vi "IT6322Control.vi"(9 "通道1":dbl, 10 "VISA resource name":refnum<visa-resource-name> caption="VISA资源名称", 11 "Sequence Context In":refnum<k7>) -> (0 "error out":errorcluster, 1 "输出":dbl, 3 "Report Text":string)   [LabVIEW 2018]
uses:
  <vilib>/Instr/_visa.llb/VISA Configure Serial Port (Instr).vi
panel:
  out "输出 3":dbl
  out "输出 2":dbl
  in  "通道3":dbl
  in  "通道2":dbl
  in  "功能":T1(ring)
  in  "error in (no error)":errorcluster caption="错误输入（无错误）"
  # "IT6322 CONTROL"
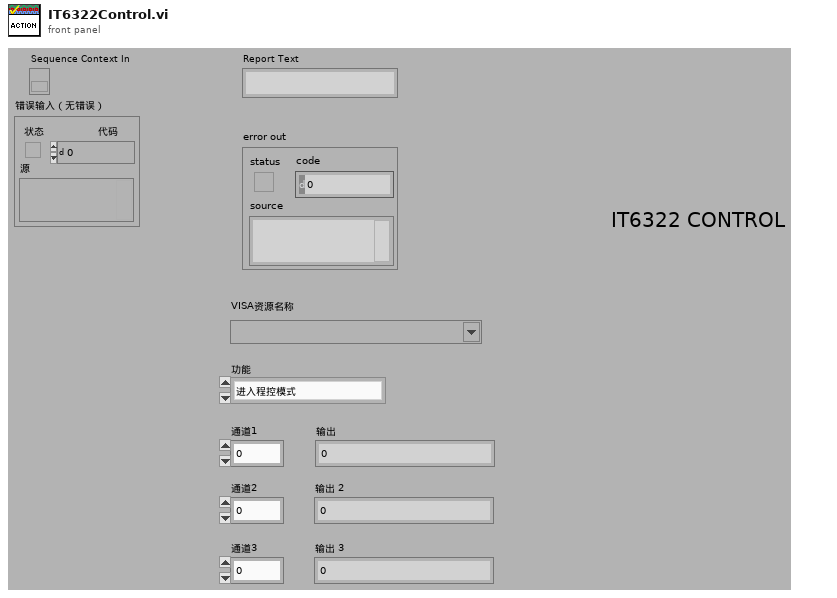
[diagram p1: front panel]
types:
  T1 = enum16{"进入程控模式", "输出ON", "输出OFF", "设置电压", "设置电流", "读取电压", "读取电流"}
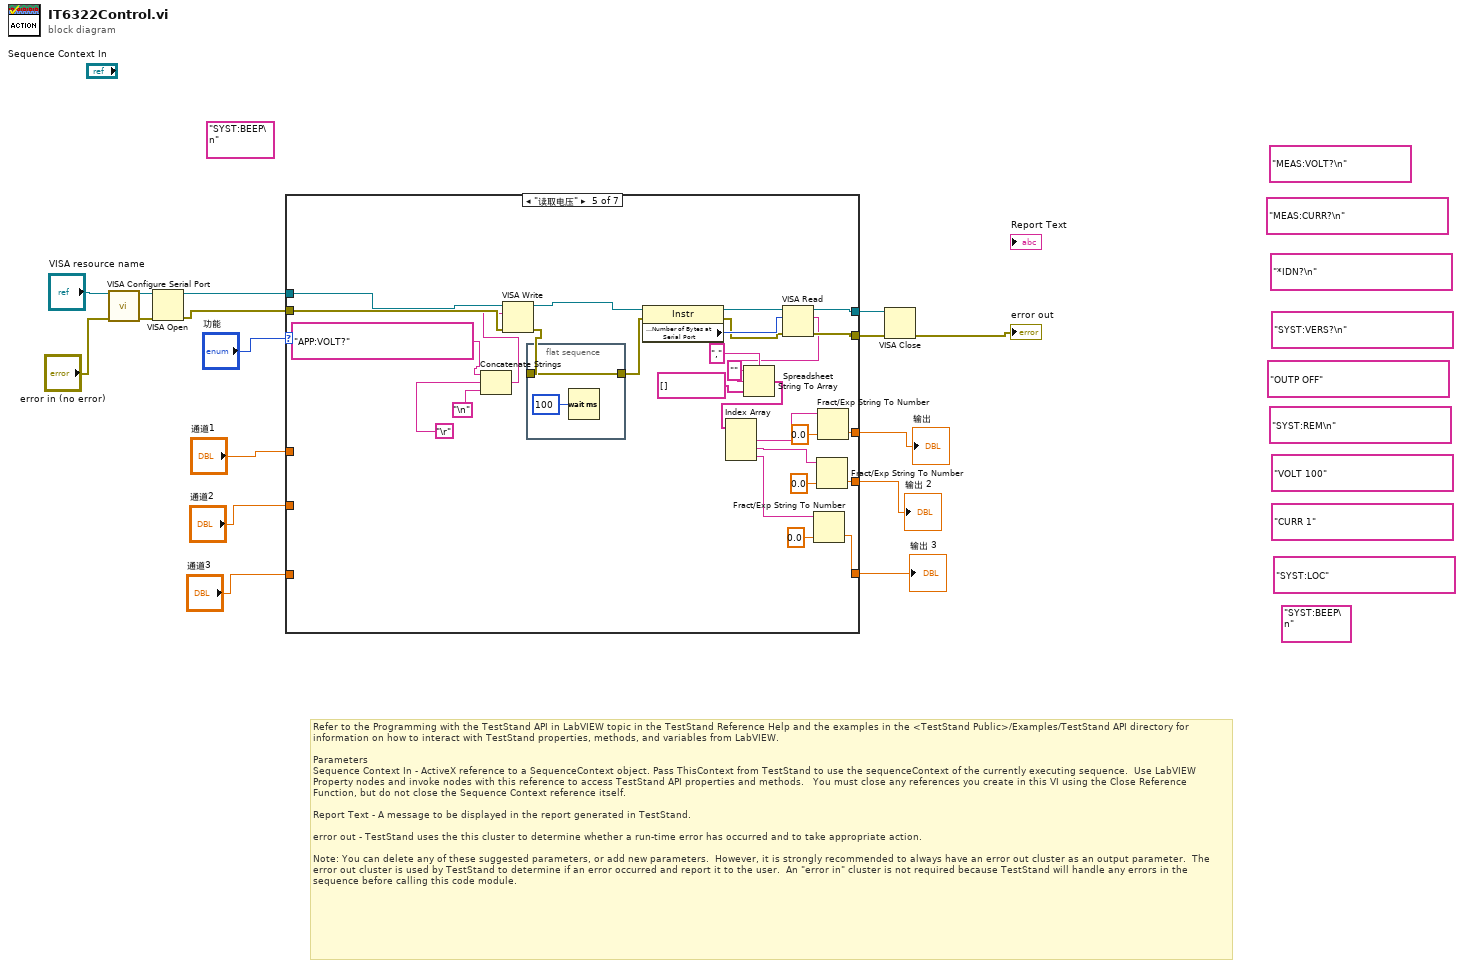
[diagram p0: block diagram]
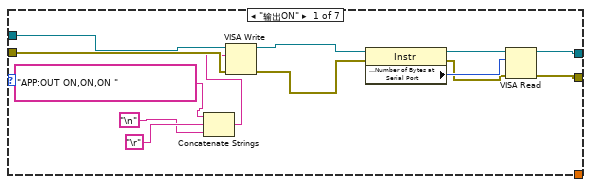
[diagram p2: hidden frame]
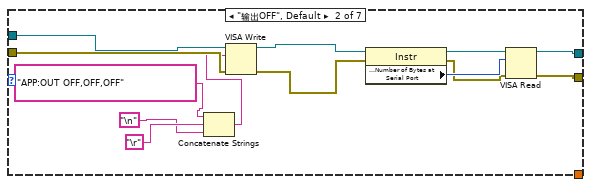
[diagram p3: hidden frame]
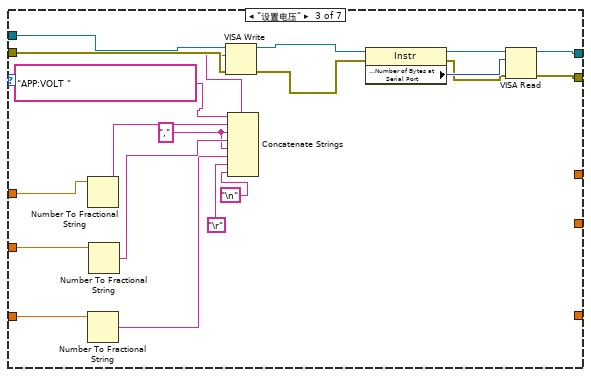
[diagram p4: hidden frame]
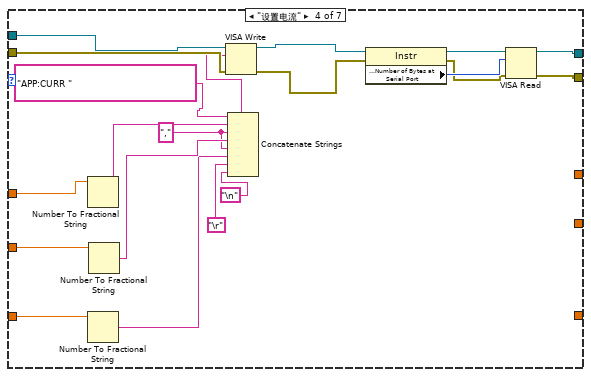
[diagram p5: hidden frame]
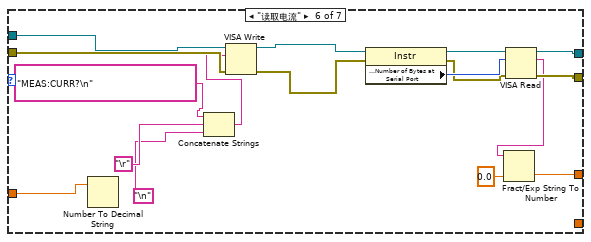
[diagram p6: hidden frame]
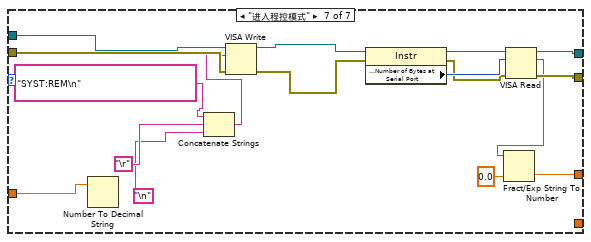
[diagram p7: hidden frame]
diagram:
  (unwired) "SYST:LOC" ("写入缓冲区")
  (unwired) "CURR 1" ("写入缓冲区")
  (unwired) "VOLT 100" ("写入缓冲区")
  (unwired) "OUTP OFF" ("写入缓冲区")
  (unwired) "SYST:REM\n" ("写入缓冲区")
  (unwired) "SYST:VERS?\n" ("写入缓冲区")
  (unwired) "*IDN?\n" ("写入缓冲区")
  (unwired) "MEAS:CURR?\n" ("写入缓冲区")
  (unwired) "MEAS:VOLT?\n" ("写入缓冲区")
  (unwired) "SYST:BEEP\n" ("写入缓冲区")
  (unwired) "SYST:BEEP\n" ("写入缓冲区")
  # "Refer to the Programming with the TestStand API in LabVIEW topic in the TestStand Reference Help and the examples in the <TestStand Public>/Examples/TestStand API directory for information on how to interact with TestStand properties, methods, and variables from LabVIEW.\n\nParameters\nSequence Context In - ActiveX reference to a SequenceContext object. Pass ThisContext from TestStand to use the sequenceContext of the currently executing sequence.  Use LabVIEW Property nodes and invoke nodes with this reference to access TestStand API properties and methods.   You must close any references you create in this VI using the Close Reference Function, but do not close the Sequence Context reference itself.\n\nReport Text - A message to be displayed in the report generated in TestStand. \n\nerror out - TestStand uses the this cluster to determine whether a run-time error has occurred and to take appropriate action.  \n\nNote: You can delete any of these suggested parameters, or add new parameters.  However, it is strongly recommended to always have an error out cluster as an output parameter.  The error out cluster is used by TestStand to determine if an error occurred and report it to the user.  An \"error in\" cluster is not required because TestStand will handle any errors in the sequence before calling this code module."
  n1 = call-poly "VISA Configure Serial Port"("VISA resource name"="VISA resource name", "error in (no error)"="error in (no error)") -> ("VISA resource name out"=w14:refnum<visa-resource-name>, "error out"=w15:errorcluster)  [unwired: 12 in]
  n2 = VISA Open(error in (no error)=w15, VISA resource name=w14) -> (VISA resource name=w13:refnum<visa-resource-name>, error out=w12:errorcluster)  [unwired: 3 in]
  n3 = case shown="\"读取电压\"" "功能" {
    tunnel: w13 -> [w29 w42 w62 w82 w110 w129 w146]
    tunnel: w12 -> [w28 w41 w61 w81 w109 w128 w145]
    tunnel: [w20 w33 w53 w73 w101 w120 w137] -> w10
    tunnel: [w19 w32 w52 w72 w100 w119 w136] -> w9
    tunnel: "通道1" -> [_ _ w48 w68 _ w116 w133]
    tunnel: [_ _ _ _ w97 w113 w130] -> w5
    tunnel: "通道2" -> [_ _ w47 w67 _ _ _]
    tunnel: "通道3" -> [_ _ w46 w66 _ _ _]
    tunnel: [_ _ _ _ w86 _ _] -> w2
    tunnel: [_ _ _ _ w85 _ _] -> w1
    frame "输出ON" {
      n4 = Concatenate Strings("APP:OUT ON,ON,ON " ("写入缓冲区"), "\r", "\n") -> (w23:string)
      n5 = VISA Write(VISA resource name=w29, write buffer=w23, error in (no error)=w28) -> (VISA resource name out=w27:refnum<visa-resource-name>, error out=w17:errorcluster)  [unwired: 1 out]
      n6 = property class="Instr"(reference=w27, error in=w17) -> (reference out=w26:refnum<visa-resource-name>, error out=w18:errorcluster, "Serial Settings:Number of Bytes at Serial Port"=w25:u32)
      n7 = VISA Read(VISA resource name=w26, byte count=w25, error in (no error)=w18) -> (VISA resource name out=w20:refnum<visa-resource-name>, error out=w19:errorcluster)  [unwired: 2 out]
    }
    frame "输出OFF", Default {
      n8 = Concatenate Strings("APP:OUT OFF,OFF,OFF" ("写入缓冲区"), "\r", "\n") -> (w36:string)
      n9 = VISA Write(VISA resource name=w42, write buffer=w36, error in (no error)=w41) -> (VISA resource name out=w40:refnum<visa-resource-name>, error out=w30:errorcluster)  [unwired: 1 out]
      n10 = property class="Instr"(reference=w40, error in=w30) -> (reference out=w39:refnum<visa-resource-name>, error out=w31:errorcluster, "Serial Settings:Number of Bytes at Serial Port"=w38:u32)
      n11 = VISA Read(VISA resource name=w39, byte count=w38, error in (no error)=w31) -> (VISA resource name out=w33:refnum<visa-resource-name>, error out=w32:errorcluster)  [unwired: 2 out]
    }
    frame "设置电压" {
      w44 = "," ("string")
      n12 = Number To Fractional String(number=w48) -> (F-format string=w49:string)  [unwired: 3 in]
      n13 = Number To Fractional String(number=w46) -> (F-format string=w43:string)  [unwired: 3 in]
      n14 = Number To Fractional String(number=w47) -> (F-format string=w45:string)  [unwired: 3 in]
      n15 = Concatenate Strings("APP:VOLT " ("写入缓冲区"), w49, w44, w45, w44, w43, "\r", "\n") -> (w56:string)
      n16 = VISA Write(VISA resource name=w62, write buffer=w56, error in (no error)=w61) -> (VISA resource name out=w60:refnum<visa-resource-name>, error out=w50:errorcluster)  [unwired: 1 out]
      n17 = property class="Instr"(reference=w60, error in=w50) -> (reference out=w59:refnum<visa-resource-name>, error out=w51:errorcluster, "Serial Settings:Number of Bytes at Serial Port"=w58:u32)
      n18 = VISA Read(VISA resource name=w59, byte count=w58, error in (no error)=w51) -> (VISA resource name out=w53:refnum<visa-resource-name>, error out=w52:errorcluster)  [unwired: 2 out]
    }
    frame "设置电流" {
      w64 = "," ("string")
      n19 = Number To Fractional String(number=w68) -> (F-format string=w69:string)  [unwired: 3 in]
      n20 = Number To Fractional String(number=w66) -> (F-format string=w63:string)  [unwired: 3 in]
      n21 = Number To Fractional String(number=w67) -> (F-format string=w65:string)  [unwired: 3 in]
      n22 = Concatenate Strings("APP:CURR " ("写入缓冲区"), w69, w64, w65, w64, w63, "\r", "\n") -> (w76:string)
      n23 = VISA Write(VISA resource name=w82, write buffer=w76, error in (no error)=w81) -> (VISA resource name out=w80:refnum<visa-resource-name>, error out=w70:errorcluster)  [unwired: 1 out]
      n24 = property class="Instr"(reference=w80, error in=w70) -> (reference out=w79:refnum<visa-resource-name>, error out=w71:errorcluster, "Serial Settings:Number of Bytes at Serial Port"=w78:u32)
      n25 = VISA Read(VISA resource name=w79, byte count=w78, error in (no error)=w71) -> (VISA resource name out=w73:refnum<visa-resource-name>, error out=w72:errorcluster)  [unwired: 2 out]
    }
    frame "读取电压" {
      n26 = Concatenate Strings("APP:VOLT?" ("写入缓冲区"), "\r", "\n") -> (w104:string)
      n27 = VISA Write(VISA resource name=w110, write buffer=w104, error in (no error)=w109) -> (VISA resource name out=w108:refnum<visa-resource-name>, error out=w95:errorcluster)  [unwired: 1 out]
      n28 = flat-sequence {
        tunnel: [w112] -> w96
        tunnel: w95 -> [w112]
        frame #0 {
          n29 = Wait (ms)(milliseconds to wait=u32 100) -> ()  [unwired: 1 out]
        }
      }
      n30 = property class="Instr"(reference=w108, error in=w96) -> (reference out=w107:refnum<visa-resource-name>, error out=w99:errorcluster, "Serial Settings:Number of Bytes at Serial Port"=w106:u32)
      n31 = VISA Read(VISA resource name=w107, byte count=w106, error in (no error)=w99) -> (VISA resource name out=w101:refnum<visa-resource-name>, read buffer=w84:string, error out=w100:errorcluster)  [unwired: 1 out]
      n32 = Spreadsheet String To Array(delimiter (Tab)=",", format string="", spreadsheet string=w84, array type (2D Dbl)=string[] []) -> (array=w90:string[])
      n33 = Index Array(array=w90) -> (element #1=w89:string, element #2=w88:string, element #3=w87:string)  [unwired: 3 in]
      n34 = Fract/Exp String To Number(string=w87, default (0 dbl)=0.0 ("默认(0 I32)")) -> (number=w85:dbl)  [unwired: 2 in, 1 out]
      n35 = Fract/Exp String To Number(string=w88, default (0 dbl)=0.0 ("默认(0 I32)")) -> (number=w86:dbl)  [unwired: 2 in, 1 out]
      n36 = Fract/Exp String To Number(string=w89, default (0 dbl)=0.0 ("默认(0 I32)")) -> (number=w97:dbl)  [unwired: 2 in, 1 out]
    }
    frame "读取电流" {
      n37 = Number To Decimal String(number=w116) -> ()  [unwired: 1 in, 1 out]
      n38 = Concatenate Strings("MEAS:CURR?\n" ("写入缓冲区"), "\r", "\n") -> (w123:string)
      n39 = VISA Write(VISA resource name=w129, write buffer=w123, error in (no error)=w128) -> (VISA resource name out=w127:refnum<visa-resource-name>, error out=w117:errorcluster)  [unwired: 1 out]
      n40 = property class="Instr"(reference=w127, error in=w117) -> (reference out=w126:refnum<visa-resource-name>, error out=w118:errorcluster, "Serial Settings:Number of Bytes at Serial Port"=w125:u32)
      n41 = VISA Read(VISA resource name=w126, byte count=w125, error in (no error)=w118) -> (VISA resource name out=w120:refnum<visa-resource-name>, read buffer=w115:string, error out=w119:errorcluster)  [unwired: 1 out]
      n42 = Fract/Exp String To Number(string=w115, default (0 dbl)=0.0 ("默认(0 I32)")) -> (number=w113:dbl)  [unwired: 2 in, 1 out]
    }
    frame "进入程控模式" {
      n43 = Number To Decimal String(number=w133) -> ()  [unwired: 1 in, 1 out]
      n44 = Concatenate Strings("SYST:REM\n" ("写入缓冲区"), "\r", "\n") -> (w140:string)
      n45 = VISA Write(VISA resource name=w146, write buffer=w140, error in (no error)=w145) -> (VISA resource name out=w144:refnum<visa-resource-name>, error out=w134:errorcluster)  [unwired: 1 out]
      n46 = property class="Instr"(reference=w144, error in=w134) -> (reference out=w143:refnum<visa-resource-name>, error out=w135:errorcluster, "Serial Settings:Number of Bytes at Serial Port"=w142:u32)
      n47 = VISA Read(VISA resource name=w143, byte count=w142, error in (no error)=w135) -> (VISA resource name out=w137:refnum<visa-resource-name>, read buffer=w132:string, error out=w136:errorcluster)  [unwired: 1 out]
      n48 = Fract/Exp String To Number(string=w132, default (0 dbl)=0.0 ("默认(0 I32)")) -> (number=w130:dbl)  [unwired: 2 in, 1 out]
    }
  }
  "输出" <- w5
  "输出 2" <- w2
  "输出 3" <- w1
  n49 = VISA Close(VISA resource name=w10, error in (no error)=w9) -> (error out=→"error out":errorcluster)
